vi "niRFUtil RFHS FIFO Flush.vi"(0 "Fifo ID":T1, 11 "error in (no error)":errorcluster) -> (4 "Fifo ID (out)":T1, 15 "error out":errorcluster)   [LabVIEW 2015, in "niRFUtil.lvlib"]
uses:
  niRFUtil.lvlib
  niRFUtil RFHS FIFO Reference.ctl
  niRFUtil RFHS FIFO.ctl
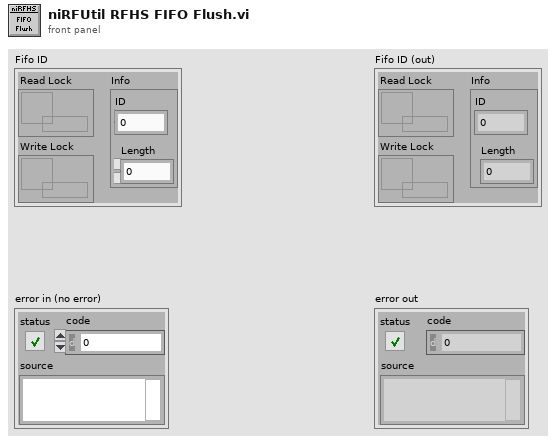
[diagram p1: front panel]
types:
  T1 = typedef "niRFUtil.lvlib/niRFUtil RFHS FIFO Reference.ctl" = cluster{"Read Lock":refnum<data-value>, "Info":T2, "Write Lock":refnum<data-value>}
  T2 = typedef "niRFUtil.lvlib/niRFUtil RFHS FIFO.ctl" = cluster{"ID":u64, "Length":u32}
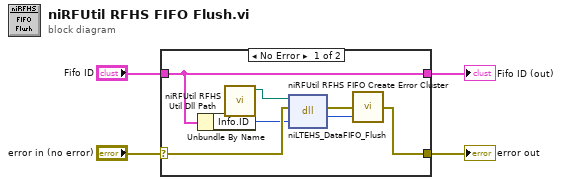
[diagram p0: block diagram]
diagram:
  n1 = case shown="No Error" "error in (no error)" {
    selector: "error in (no error)" -> [w11 w13]
    tunnel: [w6 w13] -> w3
    tunnel: "Fifo ID" -> [w8 w12]
    tunnel: [w8 w12] -> w1
    frame No Error {
      n2 = Unbundle By Name(w8) -> ("Info.ID"=w10:u64)
      n3 = call "niRFUtil RFHS Util Dll Path.vi"() -> ("Path"=w9:path)  [unwired: 7 in, 4 out]
      n4 = dll-call lib="M:/RfProtocols/RFmx/DLLs/niRFHS/trunk/2.0/dist/win32U/niRFHS_generic.dll" fn="niLTEHS_DataFIFO_Flush"(path in=w9, error in=w11, "fifoID"=w10) -> (error out=w7:errorcluster, "return type"=w5:i32)  [unwired: 2 in, 1 out]
      n5 = call "niRFUtil RFHS FIFO Create Error Cluster.vi"("error in (no error)"=w7, "fifo return value"=w5) -> ("error  out"=w6:errorcluster)  [unwired: 12 in, 1 out]
    }
    frame Error {
    }
  }
  "error out" <- w3
  "Fifo ID (out)" <- w1
